vi "LibXML_GetNodeResolvedContentStrPointer.vi"(8 "error in":errorcluster, 11 "node":u32) -> (0 "error out":errorcluster, 3 "string pointer":u32)   [LabVIEW 2019, in "Tools.lvlib" / "LibXML.lvlib"]
doc: "Gets a string pointer for the resolved content of a node input."
uses:
  LibXML.lvlib
  dll/lXMLwrap.dll
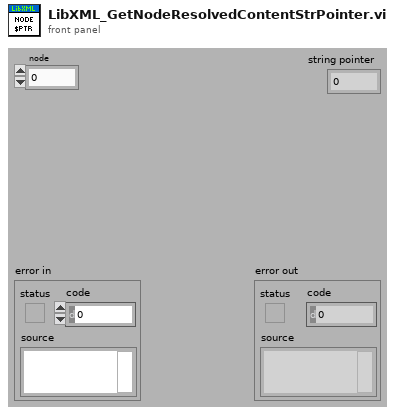
[diagram p1: front panel]
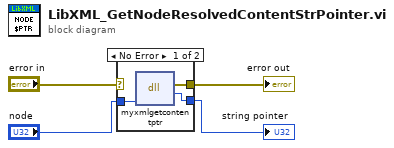
[diagram p0: block diagram]
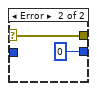
[diagram p2: hidden frame]
diagram:
  n1 = case shown="No Error" "error in" {
    selector: "error in" -> [_ w9]
    tunnel: [w5 w9] -> w3
    tunnel: "node" -> [w7 _]
    tunnel: [w6 u32 0 ("return type")] -> w1
    frame No Error {
      n2 = dll-call lib="C:/Projects/_Prywatne/MyCIT/Framework/Tools/XML/LibXML/dll/lXMLwrap.dll" fn="myxmlgetcontentptr"("node"=w7) -> (error out=w5:errorcluster, "return type"=w6:u32)  [unwired: 4 in, 1 out]
    }
    frame Error {
    }
  }
  "error out" <- w3
  "string pointer" <- w1
